vi "_Get Cell Value.vi"(8 "error in":errorcluster, 9 "Cell":refnum<k24>, 10 "Workbookpart":refnum<k24>) -> (0 "error out":errorcluster, 1 "Value Numeric":dbl, 2 "Value String":string, 4 "Type":enum16{"Void", "String", "Numeric", "Boolean"}(ring), 5 "Value Boolean":bool)   [LabVIEW 2021, in "Open Xml.lvlib"]
uses:
  Open Xml.lvlib
  D:/git/Open-Xml-LabVIEW/DocumentFormat.OpenXml.dll
  DocumentFormat.OpenXml.dll
  D:/git/Open-Xml-LabVIEW/DocumentFormat.OpenXml.Framework.dll
  DocumentFormat.OpenXml.Framework.dll
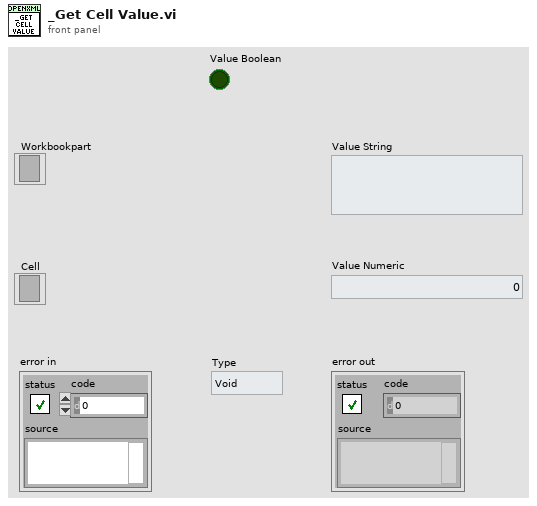
[diagram p1: front panel]
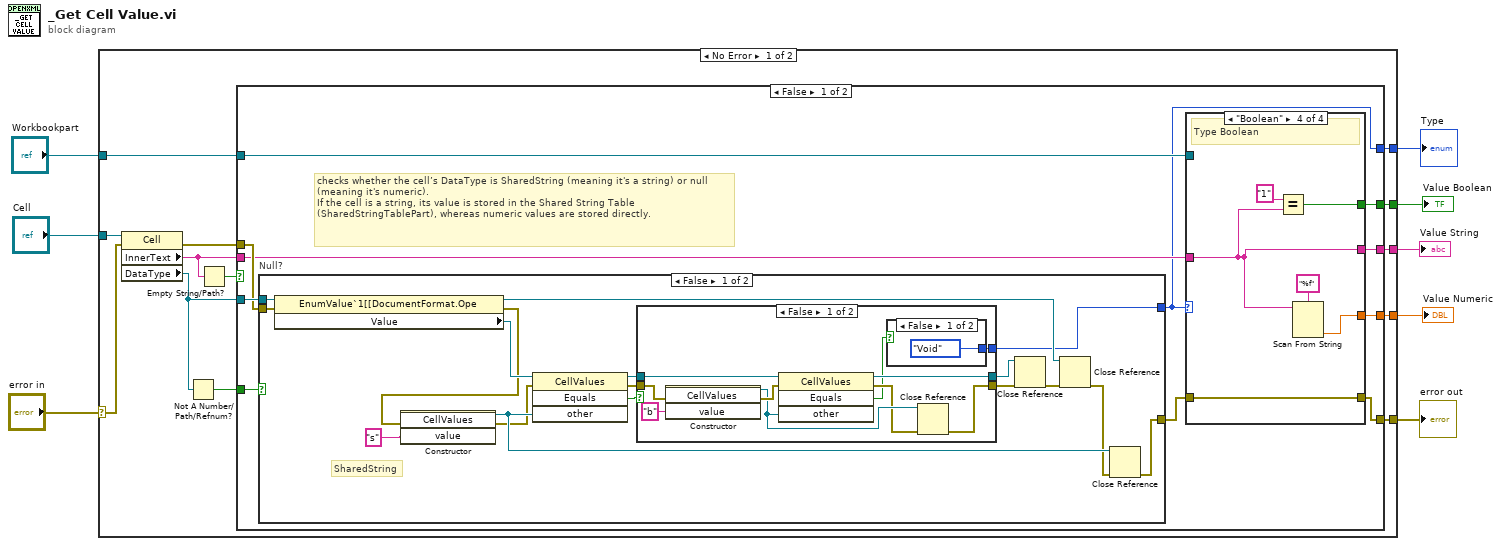
[diagram p0: block diagram]
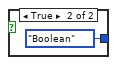
[diagram p2: hidden frame]
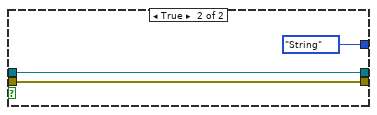
[diagram p3: hidden frame]
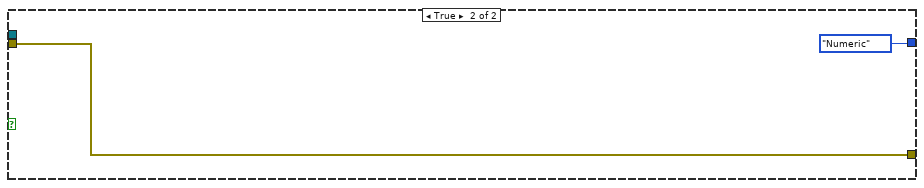
[diagram p4: hidden frame]
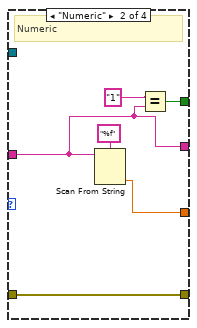
[diagram p6: hidden frame]
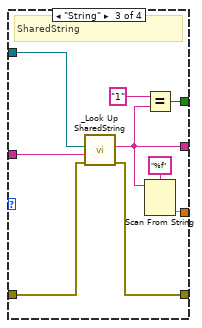
[diagram p7: hidden frame]
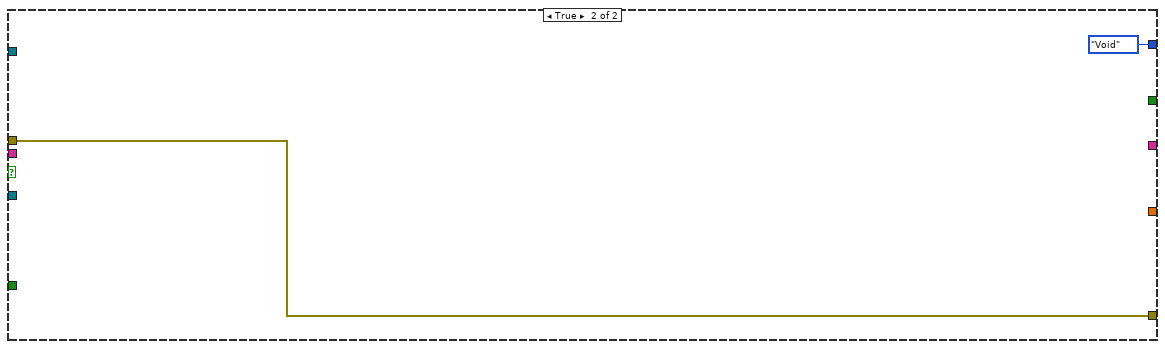
[diagram p8: hidden frame]
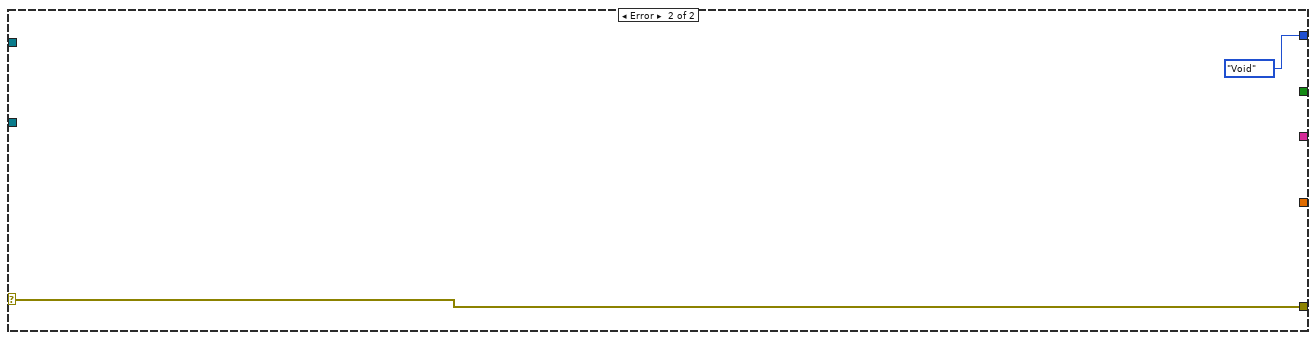
[diagram p9: hidden frame]
diagram:
  n1 = case shown="No Error" "error in" {
    selector: "error in" -> [w20 w92]
    tunnel: "Cell" -> [w21 _]
    tunnel: [w19 _] -> w6
    tunnel: "Workbookpart" -> [w18 _]
    tunnel: [w17 w92] -> w4
    tunnel: [w13 _] -> w3
    tunnel: [w12 enum16{"Void", "String", "Numeric"}."Void" ("Type")] -> w2
    tunnel: [w9 _] -> w1
    frame No Error {
      n2 = property class="Cell"(reference=w21, error in=w20) -> (error out=w14:errorcluster, "InnerText"=w11:string, "DataType"=w15:refnum<k24>)  [unwired: 1 out]
      n3 = Not A Number/Path/Refnum?(number/path/refnum=w15) -> (NaN/Path/Refnum?=w16:bool)
      n4 = Empty String/Path?(string/path=w11) -> (empty?=w10:bool)
      n5 = case shown="False" w10 {
        tunnel: [w31 _] -> w19
        tunnel: w18 -> [w30 _]
        tunnel: [w29 w90] -> w17
        tunnel: w16 -> [w28 _]
        tunnel: w15 -> [w27 _]
        tunnel: w14 -> [w26 w90]
        tunnel: [w25 _] -> w13
        tunnel: [w22 enum16{"Void", "String", "Numeric", "Boolean"}."Void" ("Type")] -> w12
        tunnel: w11 -> [w24 _]
        tunnel: [w23 _] -> w9
        frame False {
          # "checks whether the cell’s DataType is SharedString (meaning it's a string) or null (meaning it's numeric).\nIf the cell is a string, its value is stored in the Shared String Table (SharedStringTablePart), whereas numeric values are stored directly."
          n6 = case "Null?" shown="False" w28 {
            tunnel: w27 -> [w49 _]
            tunnel: [w34 w66] -> w32
            tunnel: w26 -> [w42 w66]
            tunnel: [w33 enum16{"Void", "String", "Numeric", "Boolean"}."Numeric" ("Type")] -> w22
            frame False {
              # "SharedString"
              # "Null?"
              n7 = property class="EnumValue`1[[DocumentFormat.Ope"(reference=w49, error in=w42) -> (reference out=w43:refnum<k24>, error out=w41:errorcluster, "Value"=w45:refnum<k24>)
              n8 = constructor class="CellValues"(error in=w41, "value"="s") -> (reference out=w47:refnum<k24>, error out=w40:errorcluster)  [unwired: 2 in, 2 out]
              n9 = invoke class="CellValues" method="Equals"(reference=w45, error in=w40, "other"=w47) -> (reference out=w38:refnum<k24>, error out=w37:errorcluster, "Equals"=w36:bool)  [unwired: 1 in, 1 out]
              n10 = case shown="False" w36 {
                tunnel: [w52 w64] -> w39
                tunnel: w38 -> [w59 w63]
                tunnel: w37 -> [w58 w64]
                tunnel: [w55 w63] -> w35
                tunnel: [w50 enum16{"Void", "String", "Numeric", "Boolean"}."String" ("Type")] -> w33
                frame False {
                  n11 = constructor class="CellValues"(error in=w58, "value"="b") -> (reference out=w54:refnum<k24>, error out=w57:errorcluster)  [unwired: 2 in, 2 out]
                  n12 = invoke class="CellValues" method="Equals"(reference=w59, error in=w57, "other"=w54) -> (reference out=w55:refnum<k24>, error out=w53:errorcluster, "Equals"=w51:bool)  [unwired: 1 in, 1 out]
                  n13 = case shown="False" w51 {
                    tunnel: [enum16{"Void", "String", "Numeric", "Boolean"}."Void" ("Type") enum16{"Void", "String", "Numeric", "Boolean"}."Boolean" ("Type")] -> w50
                    frame False {
                    }
                    frame True {
                    }
                  }
                  n14 = Close Reference(reference=w54, error in (no error)=w53) -> (error out=w52:errorcluster)
                }
                frame True {
                }
              }
              n15 = Close Reference(reference=w35, error in (no error)=w39) -> (error out=w46:errorcluster)
              n16 = Close Reference(reference=w43, error in (no error)=w46) -> (error out=w44:errorcluster)
              n17 = Close Reference(reference=w47, error in (no error)=w44) -> (error out=w34:errorcluster)
            }
            frame True {
            }
          }
          n18 = case "SharedString?" shown="\"Boolean\"" w22 {
            tunnel: w24 -> [_ w69 w81 w85]
            tunnel: w32 -> [w67 w71 w80 w83]
            tunnel: [_ w69 w75 w85] -> w31
            tunnel: w30 -> [_ _ w82 _]
            tunnel: [w67 w71 w79 w83] -> w29
            tunnel: [_ w73 w78 w84] -> w25
            tunnel: [_ w70 w76 w87] -> w23
            frame "Void" {
            }
            frame "Numeric" {
              # "Numeric"
              n19 = Scan From String(format string="%f", input string=w69) -> (output 1=w73:dbl)  [unwired: 3 in, 3 out]
              n20 = Equal?(x="1", y=w69) -> (x = y?=w70:bool)
            }
            frame "String" {
              # "SharedString"
              n21 = call "_Look Up SharedString.vi"("error in"=w80, "Index"=w81, "WorkbookPart"=w82) -> ("error out"=w79:errorcluster, "String Value"=w75:string)  [unwired: 7 in]
              n22 = Equal?(x="1", y=w75) -> (x = y?=w76:bool)
              n23 = Scan From String(format string="%f", input string=w75) -> (output 1=w78:dbl)  [unwired: 3 in, 3 out]
            }
            frame "Boolean" {
              # "Type Boolean"
              n24 = Equal?(x="1", y=w85) -> (x = y?=w87:bool)
              n25 = Scan From String(format string="%f", input string=w85) -> (output 1=w84:dbl)  [unwired: 3 in, 3 out]
            }
          }
        }
        frame True {
        }
      }
    }
    frame Error {
    }
  }
  "error out" <- w4
  "Value String" <- w6
  "Value Numeric" <- w3
  "Type" <- w2
  "Value Boolean" <- w1
